vi "ProjektKSP_Osika_Piotr.vi"() -> ()   [LabVIEW 2023]
panel:
  in  "Snooze time (min)":dbl=1.0
  out "Alarm light":bool
  out "Alarms":string[](array[string])
  out "Time":string
  in  "Add Alarm":bool
  in  "Off button":bool
  out "Date":string
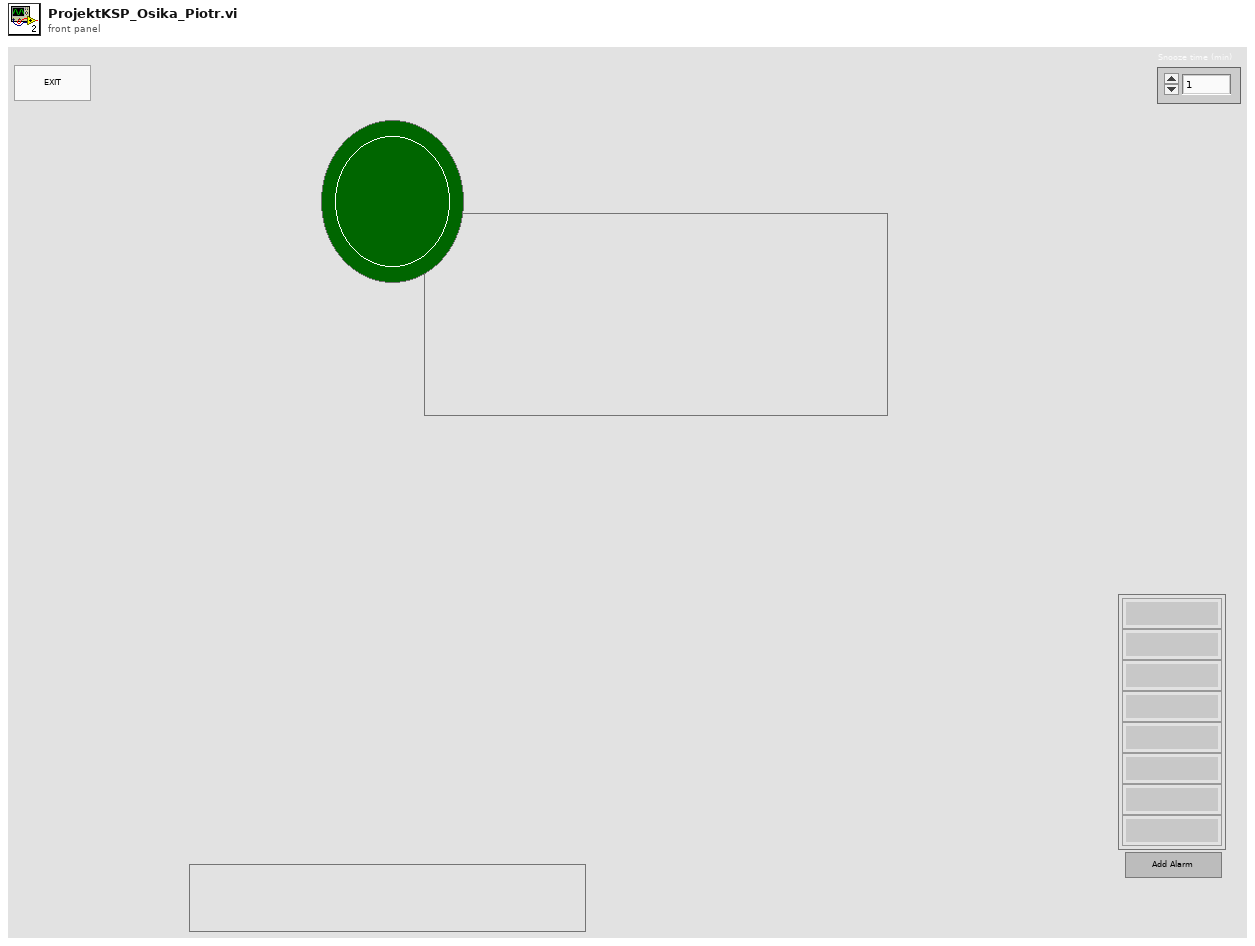
[diagram p1: front panel]
types:
  T1 = enum16{"Display", "Alarm_setup", "Compare", "Alarm"}
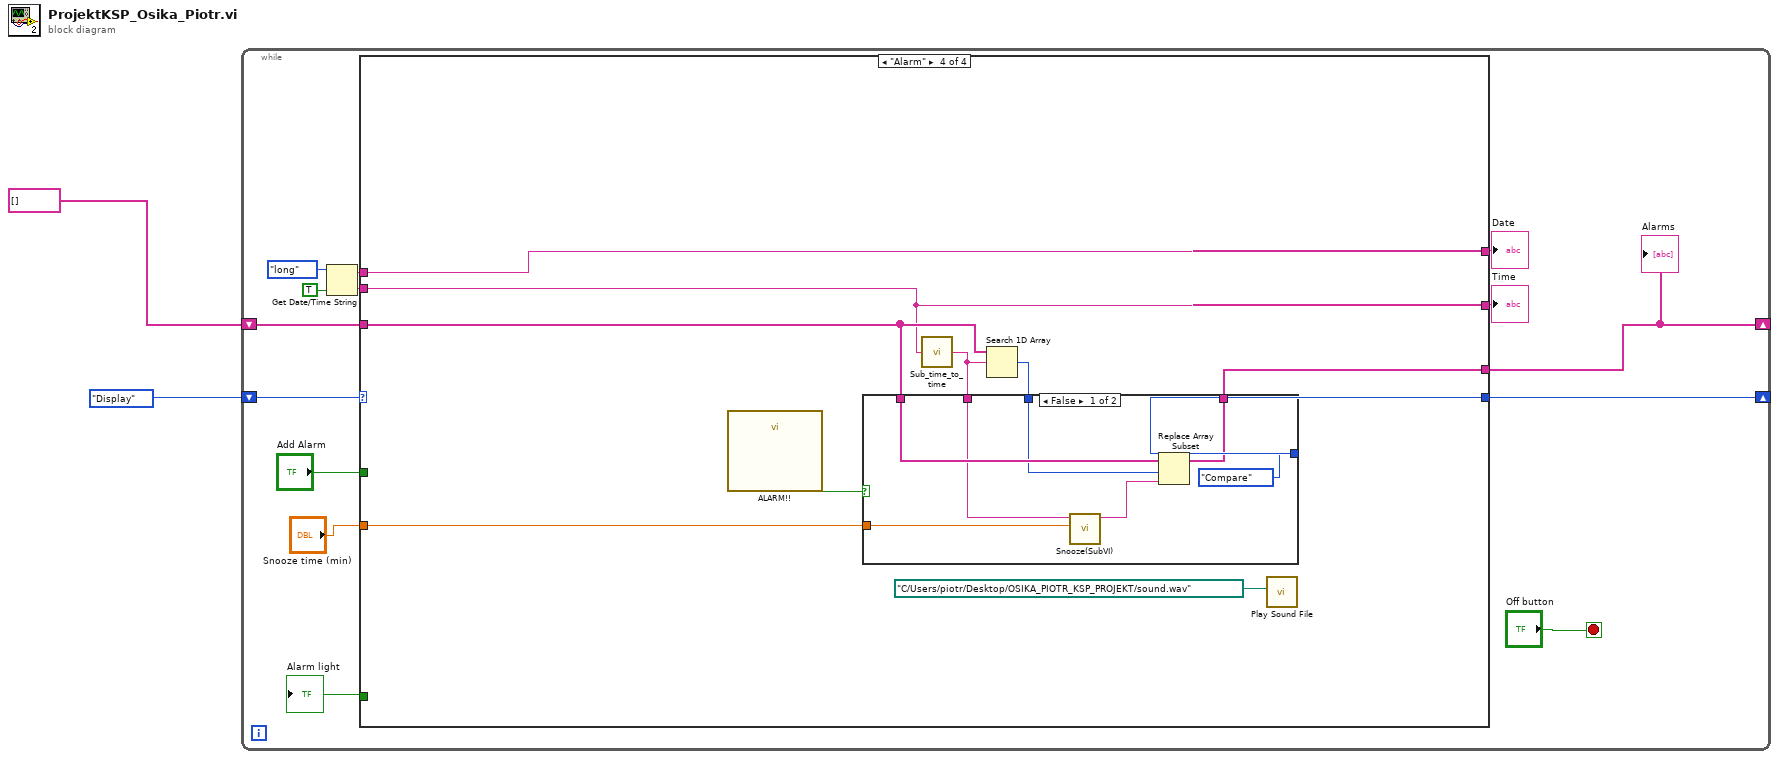
[diagram p0: block diagram]
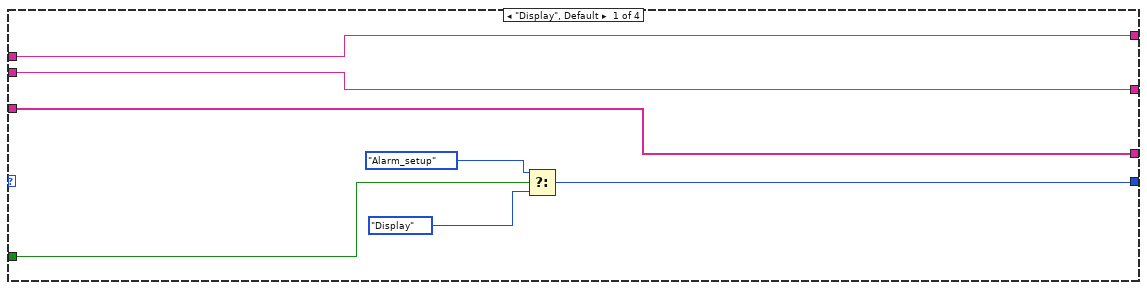
[diagram p2: hidden frame]
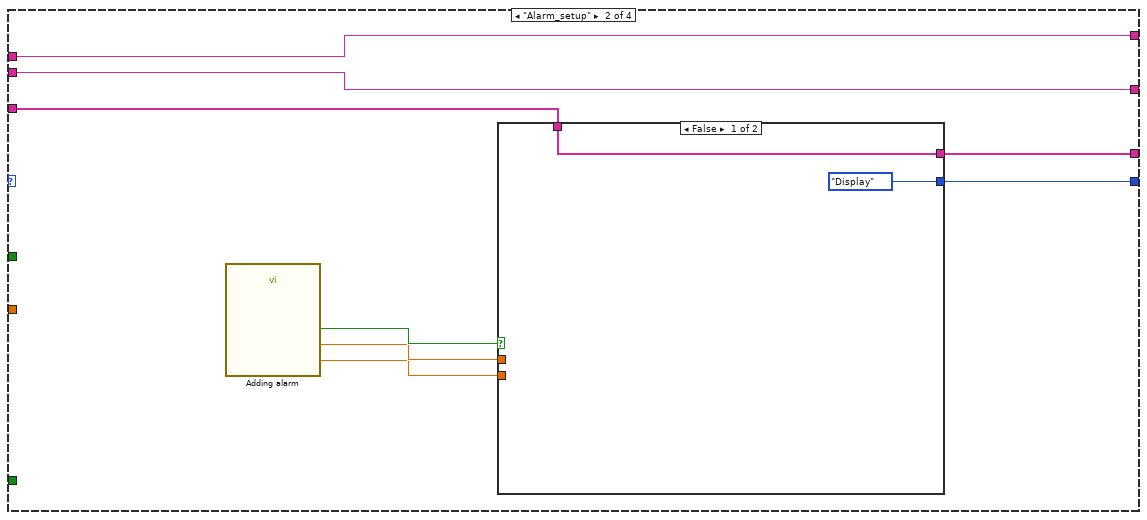
[diagram p3: hidden frame]
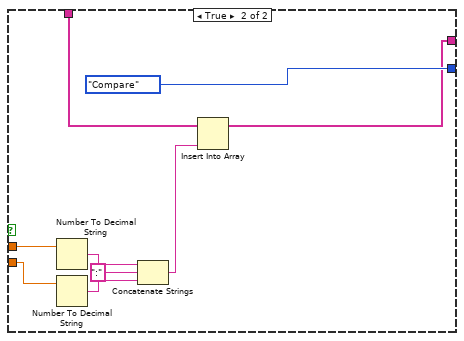
[diagram p4: hidden frame]
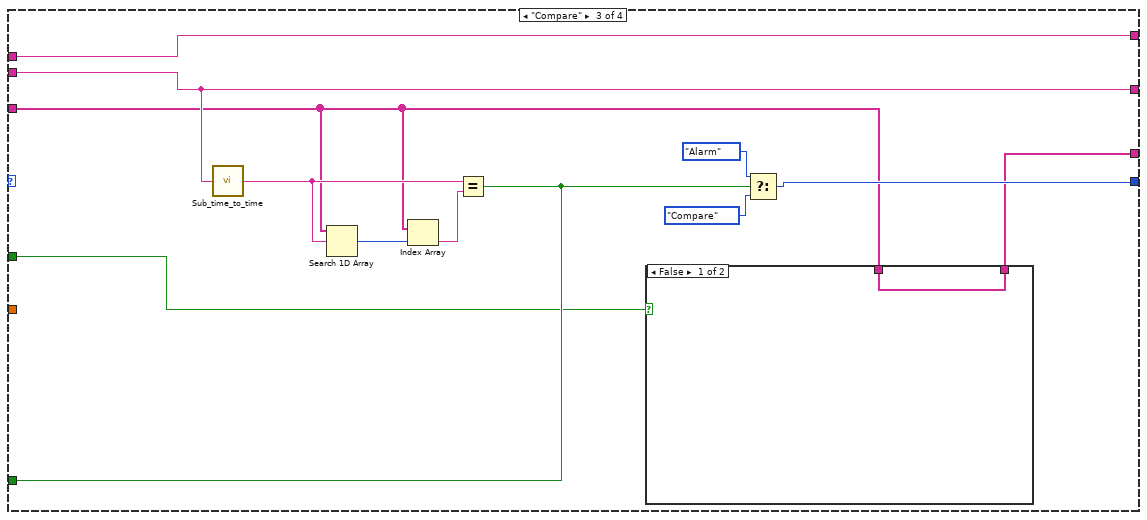
[diagram p5: hidden frame]
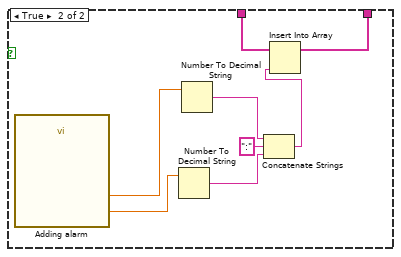
[diagram p6: hidden frame]
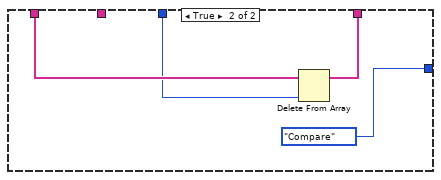
[diagram p7: hidden frame]
diagram:
  n1 = while {
    shift-right: [w6] -> _
    shift-left: T1."Display" -> [w10]
    shift-right: [w7] -> _
    shift-left: string[] [] -> [w8]
    stop <- "Off button" stop-if-true
    n2 = Get Date/Time String(date format (0)=enum16{"short", "long", "abbreviated"}."long", want seconds? (F)=TRUE) -> (date string=w14:string, time string=w13:string)  [unwired: 1 in]
    n3 = case shown="\"Alarm\"" w10 {
      tunnel: w14 -> [w22 w31 w54 w73]
      tunnel: w13 -> [w23 w30 w46 w67]
      tunnel: [w22 w31 w54 w73] -> w12
      tunnel: [w23 w30 w46 w67] -> w11
      tunnel: w8 -> [w17 w25 w44 w71]
      tunnel: [w17 w26 w50 w69] -> w7
      tunnel: [w19 w24 w51 w70] -> w6
      tunnel: "Add Alarm" -> [w18 _ w43 _]
      tunnel: [_ _ w47 _] -> w4
      tunnel: "Snooze time (min)" -> [_ _ _ w64]
      frame "Display", Default {
        n4 = Select(t=T1."Alarm_setup", s=w18, f=T1."Display") -> (s? t:f=w19:T1)
      }
      frame "Alarm_setup" {
        n5 = call "Adding alarm"() -> ("Minute"=w27:dbl, "Hour"=w28:dbl, "OK"=w29:bool)  [unwired: 16 in, 1 out]
        n6 = case shown="False" w29 {
          tunnel: w28 -> [_ w38]
          tunnel: w27 -> [_ w37]
          tunnel: w25 -> [w32 w36]
          tunnel: [w32 w35] -> w26
          tunnel: [T1."Display" T1."Compare"] -> w24
          frame False {
          }
          frame True {
            n7 = Number To Decimal String(number=w38) -> (decimal integer string=w40:string)  [unwired: 1 in]
            n8 = Number To Decimal String(number=w37) -> (decimal integer string=w39:string)  [unwired: 1 in]
            n9 = Concatenate Strings(w40, ":" ("string"), w39) -> (w34:string)
            n10 = Insert Into Array(array=w36, new element=w34) -> (w35:string[])  [unwired: 1 in]
          }
        }
      }
      frame "Compare" {
        n11 = call "Sub_time_to_time.vi"("Time"=w46) -> ("Time hh::mm"=w45:string)
        n12 = Search 1D Array(1D array=w44, element=w45) -> (index of element=w49:i32)  [unwired: 1 in]
        n13 = Index Array(array=w44, index=w49) -> (element=w48:string)
        n14 = Equal?(x=w45, y=w48) -> (x = y?=w47:bool)
        n15 = case shown="False" w43 {
          tunnel: w44 -> [w55 w58]
          tunnel: [w55 w57] -> w50
          frame False {
          }
          frame True {
            n16 = call "Adding alarm"() -> ("Minute"=w61:dbl, "Hour"=w62:dbl)  [unwired: 16 in, 2 out]
            n17 = Number To Decimal String(number=w61) -> (decimal integer string=w59:string)  [unwired: 1 in]
            n18 = Number To Decimal String(number=w62) -> (decimal integer string=w60:string)  [unwired: 1 in]
            n19 = Concatenate Strings(w60, ":" ("string"), w59) -> (w56:string)
            n20 = Insert Into Array(array=w58, new element=w56) -> (w57:string[])  [unwired: 1 in]
          }
        }
        n21 = Select(t=T1."Alarm", s=w47, f=T1."Compare") -> (s? t:f=w51:T1)
      }
      frame "Alarm" {
        n22 = call "ALARM!!"() -> ("OK"=w72:bool)  [unwired: 18 in, 1 out]
        n23 = call "Sub_time_to_time.vi"("Time"=w67) -> ("Time hh::mm"=w65:string)
        n24 = Search 1D Array(1D array=w71, element=w65) -> (index of element=w66:i32)  [unwired: 1 in]
        n25 = case shown="False" w72 {
          tunnel: w71 -> [w77 w83]
          tunnel: [w78 w82] -> w69
          tunnel: [T1."Compare" T1."Compare"] -> w70
          tunnel: w66 -> [w76 w81]
          tunnel: w65 -> [w75 _]
          tunnel: w64 -> [w74 _]
          frame False {
            n26 = call "Snooze(SubVI).vi"("snooze"=w74, "Time hh::mm"=w75) -> ("Time hh::mm + snooze"=w79:string)  [unwired: 9 in]
            n27 = Replace Array Subset(array=w77, new element=w79, index=w76) -> (w78:string[])
          }
          frame True {
            n28 = Delete From Array(array=w83, index=w81) -> (array with subset deleted=w82:string[])  [unwired: 1 in, 1 out]
          }
        }
        n29 = call <vilib>:"Play Sound File.vi"("path"=path "C:/Users/piotr/Desktop/OSIKA_PIOTR_KSP_PROJEKT/sound.wav") -> ()  [unwired: 9 in, 2 out]
      }
    }
    "Date" <- w12
    "Time" <- w11
    "Alarms" <- w7
    "Alarm light" <- w4
  }
